vi "ELIMINA_FONDO_SIN BUFFER(subVI).vi"(6 "Image Type":T1=4 items=["Grayscale (U8)", "Grayscale (I16)", "Grayscale (SGL)", "Complex (CSG)", "RGB (U32)", "HSL (U32)", "RGB (U64)"], 8 "error in":errorcluster, 9 "Backgroud In":T2, 11 "Image In":T2) -> (0 "error out":errorcluster, 2 "Image 1 Add 2":T2, 5 "Subtract 2 Back-ImageIn":T2, 7 "Subtrack 1 ImageIn-back":T2)   [LabVIEW 2011]
doc: "Elimina el fondo: a nueva imagen le resta el fondo y al fondo le resta la nueva, y el resultado lo suma.\nCualquier nuevo pixel de la nueva imagen que no estuviera en el fondo es detectado."
uses:
  IMAQ Image.ctl
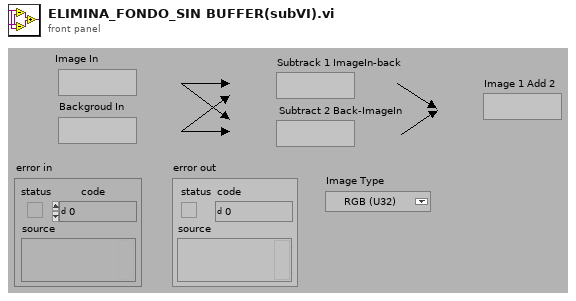
[diagram p1: front panel]
types:
  T1 = typedef "Image Type" = u32
  T2 = typedef "IMAQ Image.ctl" = cluster{string, u32}
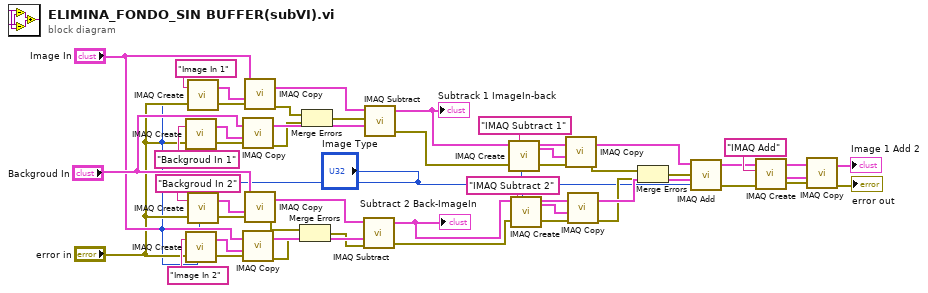
[diagram p0: block diagram]
diagram:
  n1 = call "IMAQ Create.vi"("Image Name"="Backgroud In 1", "Image Type"="Image Type", "error in (no error)"="error in") -> ("New Image"=w27:T2, "error out"=w26:errorcluster)  [unwired: 1 in, 1 out]
  n2 = call "IMAQ Create.vi"("Image Name"="Image In 2", "Image Type"="Image Type", "error in (no error)"="error in") -> ("New Image"=w35:T2, "error out"=w33:errorcluster)  [unwired: 1 in, 1 out]
  n3 = call "IMAQ Create.vi"("Image Name"="Image In 1", "Image Type"="Image Type", "error in (no error)"="error in") -> ("New Image"=w23:T2, "error out"=w22:errorcluster)  [unwired: 1 in, 1 out]
  n4 = call "IMAQ Create.vi"("Image Name"="Backgroud In 2", "Image Type"="Image Type", "error in (no error)"="error in") -> ("New Image"=w34:T2, "error out"=w32:errorcluster)  [unwired: 1 in, 1 out]
  n5 = call "IMAQ Copy"("error in (no error)"=w26, "Image Dst"=w27, "Image Src"="Backgroud In") -> ("error out"=w14:errorcluster, "Image Dst Out"=w24:T2)  [unwired: 3 out]
  n6 = call "IMAQ Copy"("error in (no error)"=w33, "Image Dst"=w35, "Image Src"="Image In") -> ("error out"=w10:errorcluster, "Image Dst Out"=w29:T2)  [unwired: 3 out]
  n7 = call "IMAQ Copy"("error in (no error)"=w22, "Image Dst"=w23, "Image Src"="Image In") -> ("error out"=w15:errorcluster, "Image Dst Out"=w20:T2)  [unwired: 3 out]
  n8 = call "IMAQ Copy"("error in (no error)"=w32, "Image Dst"=w34, "Image Src"="Backgroud In") -> ("error out"=w11:errorcluster, "Image Dst Out"=w28:T2)  [unwired: 3 out]
  n9 = Merge Errors(w11, w10) -> (w12:errorcluster)
  n10 = Merge Errors(w15, w14) -> (w13:errorcluster)
  n11 = call "IMAQ Subtract"("Image Src A"=w28, "Image Src B"=w29, "error in (no error)"=w12) -> ("Image Dst Out"=w42:T2, "error out"=w9:errorcluster)  [unwired: 2 in, 2 out]
  "Subtract 2 Back-ImageIn" <- w42
  n12 = call "IMAQ Subtract"("Image Src A"=w20, "Image Src B"=w24, "error in (no error)"=w13) -> ("Image Dst Out"=w37:T2, "error out"=w8:errorcluster)  [unwired: 2 in, 2 out]
  "Subtrack 1 ImageIn-back" <- w37
  n13 = call "IMAQ Create.vi"("Image Name"="IMAQ Subtract 1", "Image Type"="Image Type", "error in (no error)"=w8) -> ("New Image"=w45:T2, "error out"=w39:errorcluster)  [unwired: 1 in, 1 out]
  n14 = call "IMAQ Create.vi"("Image Name"="IMAQ Subtract 2", "Image Type"="Image Type", "error in (no error)"=w9) -> ("New Image"=w43:T2, "error out"=w41:errorcluster)  [unwired: 1 in, 1 out]
  n15 = call "IMAQ Copy"("error in (no error)"=w39, "Image Dst"=w45, "Image Src"=w37) -> ("error out"=w6:errorcluster, "Image Dst Out"=w38:T2)  [unwired: 3 out]
  n16 = call "IMAQ Copy"("error in (no error)"=w41, "Image Dst"=w43, "Image Src"=w42) -> ("error out"=w5:errorcluster, "Image Dst Out"=w40:T2)  [unwired: 3 out]
  n17 = Merge Errors(w6, w5) -> (w7:errorcluster)
  n18 = call "IMAQ Add"("Image Src A"=w38, "Image Src B"=w40, "error in (no error)"=w7) -> ("Image Dst Out"=w36:T2, "error out"=w18:errorcluster)  [unwired: 2 in, 2 out]
  n19 = call "IMAQ Create.vi"("Image Name"="IMAQ Add", "Image Type"="Image Type", "error in (no error)"=w18) -> ("New Image"=w47:T2, "error out"=w17:errorcluster)  [unwired: 1 in, 1 out]
  n20 = call "IMAQ Copy"("error in (no error)"=w17, "Image Dst"=w47, "Image Src"=w36) -> ("error out"=→"error out":errorcluster, "Image Dst Out"=→"Image 1 Add 2":T2)  [unwired: 3 out]
